vi "Gas Flow Panels.vi"() -> ()   [LabVIEW 2011]
panel:
  in  "Radio Buttons":T1(radio)
  in  "stop":bool
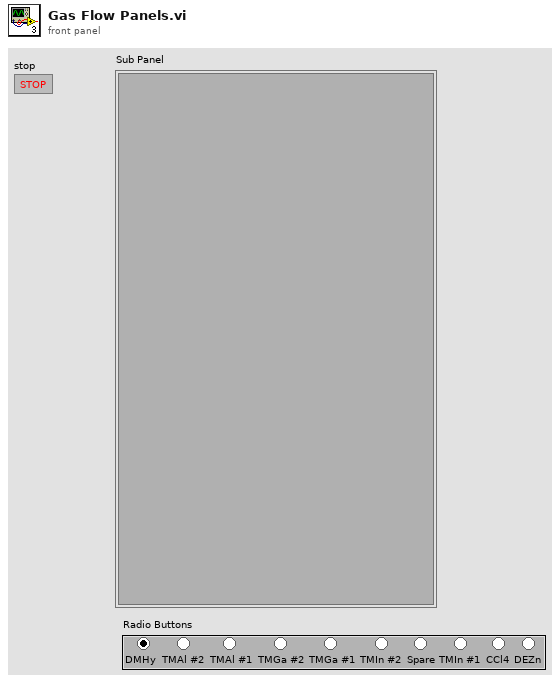
[diagram p1: front panel]
types:
  T1 = enum32{"DMHy", "TMAl #2", "TMAl #1", "TMGa #2", "TMGa #1", "TMIn #2", "Spare", "TMIn #1", "CCl4", "DEZn"}
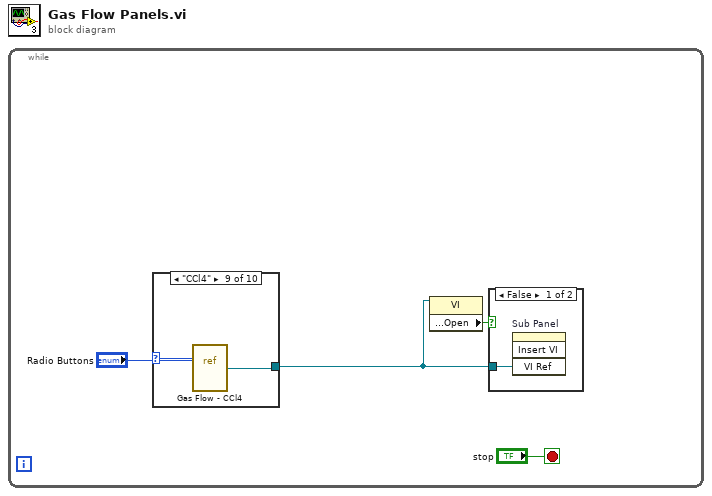
[diagram p0: block diagram]
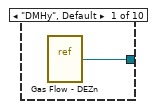
[diagram p2: hidden frame]
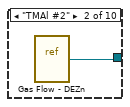
[diagram p3: hidden frame]
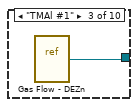
[diagram p4: hidden frame]
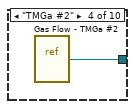
[diagram p5: hidden frame]
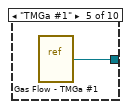
[diagram p6: hidden frame]
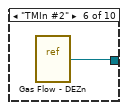
[diagram p7: hidden frame]
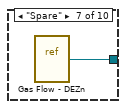
[diagram p8: hidden frame]
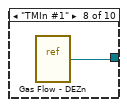
[diagram p9: hidden frame]
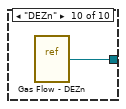
[diagram p10: hidden frame]
diagram:
  n1 = while {
    stop <- "stop" stop-if-true
    n2 = case shown="\"CCl4\"" "Radio Buttons" {
      tunnel: [w5 w6 w7 w8 w9 w10 w11 w12 w13 w14] -> w1
      frame "DMHy", Default {
        n3 = vi-ref "Gas Flow - DEZn.vi"() -> (w5:refnum<vi>)
      }
      frame "TMAl #2" {
        n4 = vi-ref "Gas Flow - DEZn.vi"() -> (w6:refnum<vi>)
      }
      frame "TMAl #1" {
        n5 = vi-ref "Gas Flow - DEZn.vi"() -> (w7:refnum<vi>)
      }
      frame "TMGa #2" {
        n6 = vi-ref "Gas Flow - TMGa #2.vi"() -> (w8:refnum<vi>)
      }
      frame "TMGa #1" {
        n7 = vi-ref "Gas Flow - TMGa #1.vi"() -> (w9:refnum<vi>)
      }
      frame "TMIn #2" {
        n8 = vi-ref "Gas Flow - DEZn.vi"() -> (w10:refnum<vi>)
      }
      frame "Spare" {
        n9 = vi-ref "Gas Flow - DEZn.vi"() -> (w11:refnum<vi>)
      }
      frame "TMIn #1" {
        n10 = vi-ref "Gas Flow - DEZn.vi"() -> (w12:refnum<vi>)
      }
      frame "CCl4" {
        n11 = vi-ref "Gas Flow - CCl4.vi"() -> (w13:refnum<vi>)
      }
      frame "DEZn" {
        n12 = vi-ref "Gas Flow - DEZn.vi"() -> (w14:refnum<vi>)
      }
    }
    n13 = property class="VI"(reference=w1) -> ("Front Panel.Open"=w3:bool)  [unwired: 1 in, 2 out]
    n14 = case shown="False" w3 {
      tunnel: w1 -> [w15 _]
      frame False {
        n15 = invoke on="Sub Panel" class="SubPanel" method="Insert VI"("VI Ref"=w15) -> ()  [unwired: 3 in, 4 out]
      }
      frame True {
      }
    }
  }
